vi "Measurement Logic.vi"() -> ()   [LabVIEW 2021, in "Single Tone_Class D Amplifier.lvlib"]
uses:
  Single Tone_Class D Amplifier.lvlib
  Measurement Results.ctl
  <vilib>/PDM Acquisition Toolkit/shared/controls/clock mode.ctl
  <vilib>/PDM Acquisition Toolkit/shared/PDM Shared.lvlib
  <vilib>/PDM Acquisition Toolkit/host/API/PDM Acquisition Toolkit.lvlib
  <vilib>/PDM Acquisition Toolkit/shared/controls/Digital Edge.ctl
  <vilib>/PDM Acquisition Toolkit/shared/controls/PCM Frame Sync Control.ctl
  <vilib>/PDM Acquisition Toolkit/shared/controls/PCM Data Justification.ctl
  <vilib>/PDM Acquisition Toolkit/shared/controls/PCM Bit Endianness.ctl
  <vilib>/PDM Acquisition Toolkit/shared/controls/PCM Data Format Configuration.ctl
  <vilib>/PDM Acquisition Toolkit/host/API/Public/Function Generator/Configure Custom Signal (N Ch) - PCM Output Task.vi
  shared/controls/units - snr.ctl
  shared/controls/audio controls.lvlib
  shared/controls/units - ratio.ctl
  shared/controls/units settings.ctl
  shared/controls/weighting filter.ctl
  shared/controls/highpass filter.ctl
  shared/controls/lowpass filter.ctl
  shared/controls/audio filter settings.ctl
  shared/controls/single tone audio measurement settings.ctl
  shared/controls/digital audio protocol/digital audio protocol controls.lvlib
  <vilib>/Waveform/WDTOps.llb/WDT Get Waveform Subset DBL.vi
  <vilib>/DAQmx/read.llb/DAQmx Read (Analog 1D Wfm NChan NSamp).vi
  <vilib>/DAQmx/configure/timing.llb/DAQmx Timing (Sample Clock).vi
  <vilib>/DAQmx/create/channels.llb/DAQmx Create Channel (AI-Voltage-Basic).vi
  Measurement Configuration.ctl
  <vilib>/MeasurementLink/MeasurementLink Measurement Server/Measure Call Context/Measure Call Context.lvclass
  shared/controls/digital output level units.ctl
  shared/controls/single tone audio measurements.ctl
panel:
  out "names out":string[](array[string])
  out "results":T1[](array[typedef])
  out "Spectrum":cluster{"x0":dbl, "dx":dbl, "magnitude":dbl[]}[](graph)
  out "Waveform Graph":waveform(dbl)[](graph)=[{"t0"=timestamp(3785336549.595634 s since 1904-01-01), "dt"=1.9531249997269942e-05, "Y"=array[12800 elements], "attributes"=variant("NI_ChannelName"=variant(string "PXI1Slot4/ai0"), "NI_UnitDescription"=variant(string "Volts"))}]
  out "Bit Clock Rate":sgl=3072000.0 format="%#_6pHz"
  out "measure call context out":refnum<class "Measure Call Context.lvclass">
  in  "measure call context in":refnum<class "Measure Call Context.lvclass">
  out "measurement results":T2={"channel names"=[], "frequency (Hz)"=[], "amplitude (Vrms)"=[], "amplitude (dBFS)"=[], "phase (deg)"=[], "SNR"=[], "THD+N"=[], "THD"=[], "dynamic range (dB)"=[], "gain"=[], "SFDR (dBc)"=[], "output power (W)"=[], "wfm - t0"=0.0, "wfm - dt"=1.9531249997269942e-05, "wfm - data"=array[12800 elements], "fft - f0"=0.0, "fft - df"=4.000000000559116, "fft - data"=array[6400 elements]}
  in  "measurement configuration":T3={"digital serial cfg file"="", "digital channel list"="7821\\PCMo 8", "master clock channel list"="7821\\PCMo 0", "signal frequency"=1000.0, "output level"=1.0, "output level units"=enum."% FS", "output range (pk-pk)"=15.0, "load impedance"=4.0, "signal phase"=0.0, "acq sampling rate"=51200.0, "min measurement cycles"=20, "min measurement time (s)"=0.1, "min settling cycles"=0, "min settling time (s)"=0.005, "acq channel"="PXI1Slot4/ai0", "band start"=20.0, "band stop"=20000.0, "weighting filter"=enum."Linear", "lowpass filter"=enum."No filter", "highpass filter"=enum."DC", "SNR units"=enum."dB", "THD+N units"=enum."dB", "THD units"=enum."dB", "gain units"=enum."dB"} {"acq sampling rate" format="%#_6p"}
  out "error out":errorcluster
  in  "error in":errorcluster
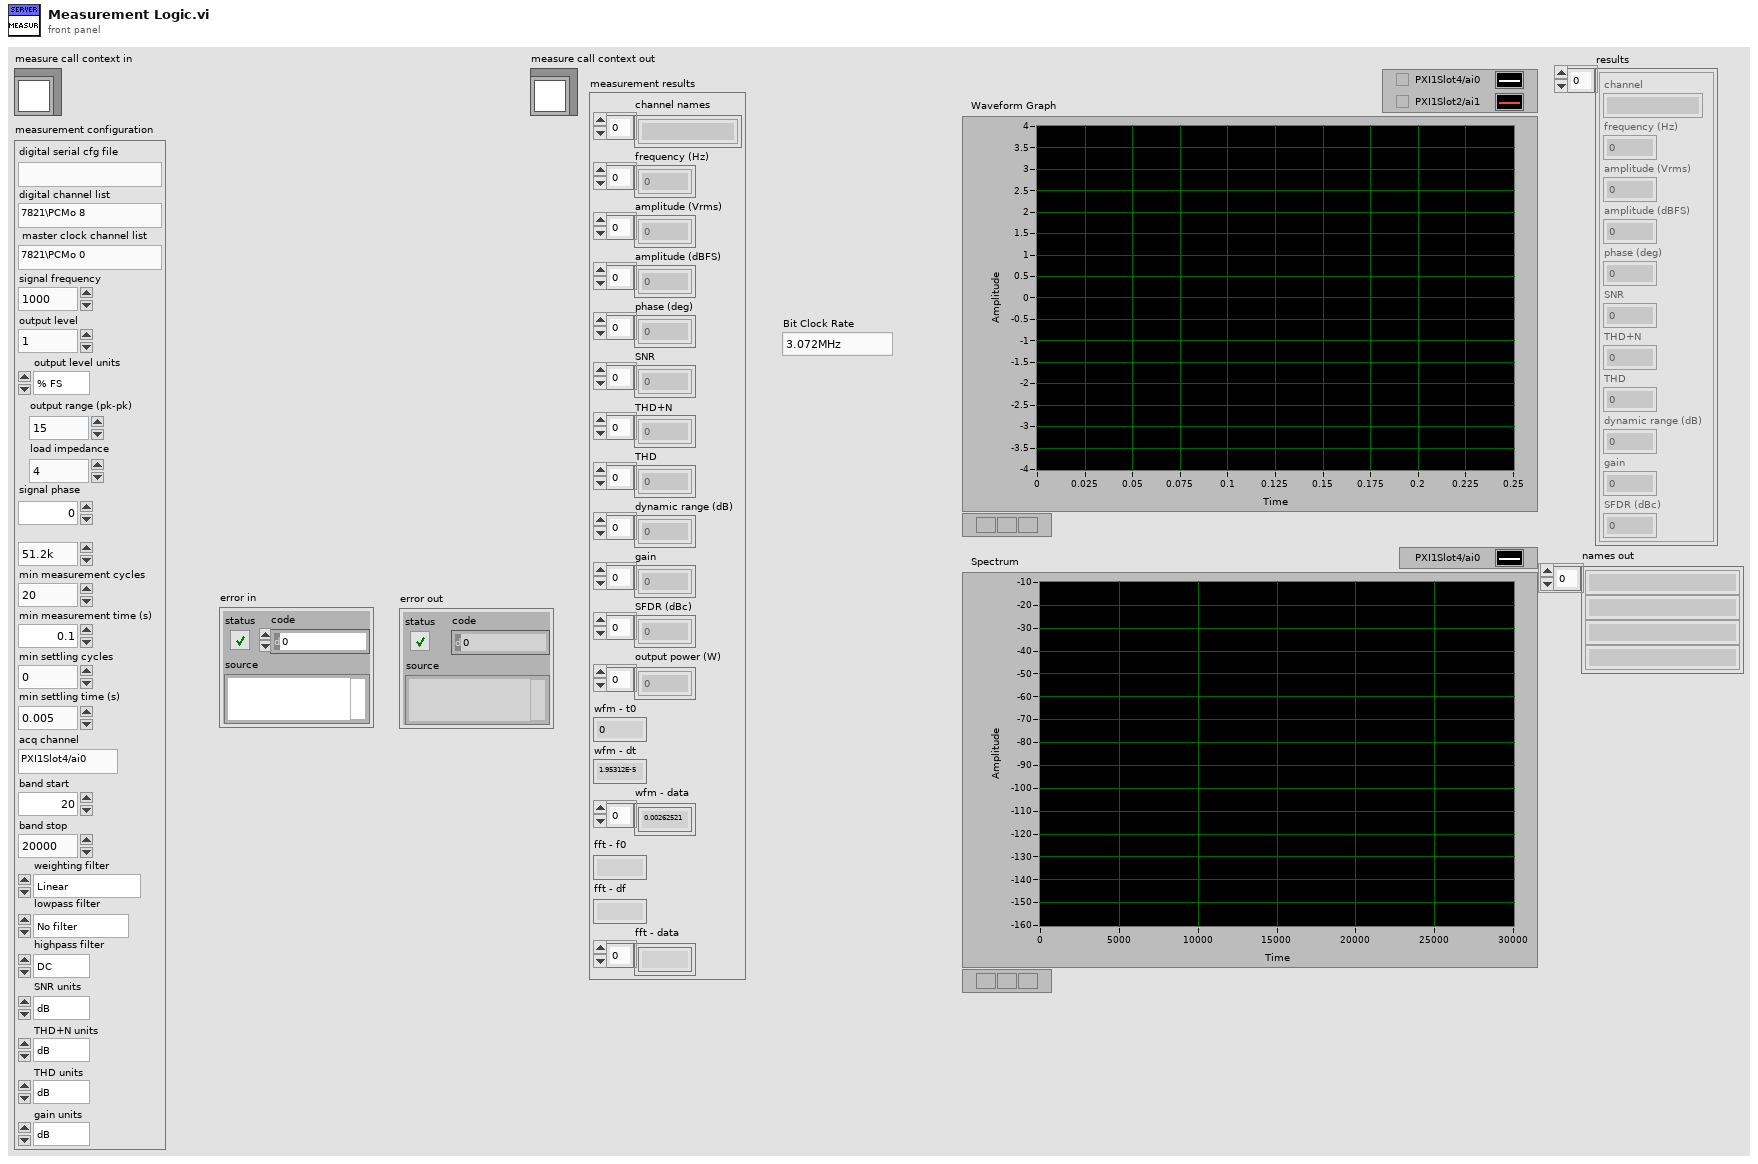
[diagram p1: front panel]
types:
  T1 = typedef "audio controls.lvlib/single tone audio measurements.ctl" = cluster{"channel":string, "frequency (Hz)":dbl, "amplitude (Vrms)":dbl, "amplitude (dBFS)":dbl, "phase (deg)":dbl, "SNR":dbl, "THD+N":dbl, "THD":dbl, "dynamic range (dB)":dbl, "gain":dbl, "SFDR (dBc)":dbl}
  T2 = typedef "Single Tone_Class D Amplifier.lvlib/Measurement Results.ctl" = cluster{"channel names":string[], "frequency (Hz)":dbl[], "amplitude (Vrms)":dbl[], "amplitude (dBFS)":dbl[], "phase (deg)":dbl[], "SNR":dbl[], "THD+N":dbl[], "THD":dbl[], "dynamic range (dB)":dbl[], "gain":dbl[], "SFDR (dBc)":dbl[], "output power (W)":dbl[], "wfm - t0":dbl, "wfm - dt":dbl, "wfm - data":dbl[], "fft - f0":dbl, "fft - df":dbl, "fft - data":dbl[]}
  T3 = typedef "Single Tone_Class D Amplifier.lvlib/Measurement Configuration.ctl" = cluster{"digital serial cfg file":string, "digital channel list":string, "master clock channel list":string, "signal frequency":dbl, "output level":dbl, "output level units":T4, "output range (pk-pk)":dbl, "load impedance":dbl, "signal phase":dbl, "acq sampling rate":dbl, "min measurement cycles":u32, "min measurement time (s)":dbl, "min settling cycles":u32, "min settling time (s)":dbl, "acq channel":string, "band start":dbl, "band stop":dbl, "weighting filter":T5, "lowpass filter":T6, "highpass filter":T7, "SNR units":T8, "THD+N units":T9, "THD units":T9, "gain units":T9}
  T4 = typedef "audio controls.lvlib/digital output level units.ctl" = enum32{"% FS", "dBFS", "V"}
  T5 = typedef "weighting filter.ctl" = enum32{"Linear", "A-weighting", "B-weighting", "C-weighting"}
  T6 = typedef "lowpass filter.ctl" = enum32{"No filter", "AES17 20kHz", "AES17 40kHz"}
  T7 = typedef "highpass filter.ctl" = enum32{"DC", "AC"}
  T8 = typedef "audio controls.lvlib/units - snr.ctl" = enum32{"dB", "x/y"}
  T9 = typedef "audio controls.lvlib/units - ratio.ctl" = enum32{"dB", "%", "x/y"}
  T10 = typedef "audio controls.lvlib/units settings.ctl" = cluster{"SNR units":T8, "THD+N units":T9, "THD units":T9, "gain units":T9}
  T11 = typedef "audio filter settings.ctl" = cluster{"weighting filter":T5, "highpass filter":T7, "lowpass filter ":T6}
  T12 = typedef "single tone audio measurement settings.ctl" = cluster{"Band start":dbl, "Band stop":dbl, "Amplitude":dbl, "Frequency":dbl, "Full scale range":dbl}
  T13 = typedef "PDM Shared.lvlib/PCM Data Format Configuration.ctl" = cluster{"Frame Sync Edge for Channel 0":T14, "Channel Count Per Frame":u8, "Channel Length":u16, "Bit Depth":u8, "Channel 0 Offset":u16, "Endianness":T15, "Data Justification":T16}
  T14 = typedef "PDM Shared.lvlib/Digital Edge.ctl" = enum8{"Rising", "Falling"}
  T15 = typedef "PDM Shared.lvlib/PCM Bit Endianness.ctl" = enum16{"MSB First", "LSB First"}
  T16 = typedef "PDM Shared.lvlib/PCM Data Justification.ctl" = enum16{"Left Justified", "Right Justified"}
  T17 = typedef "PDM Shared.lvlib/PCM Frame Sync Control.ctl" = cluster{"Frame Length":u16, "Frame Sync Pulse Width":u16, "Bit Clock Edge  Sync":T14}
  T18 = typedef "PDM Shared.lvlib/clock mode.ctl" = enum16{"divided clock", "DDS"}
  T19 = typedef "digital audio protocol controls.lvlib/digital audio protocol settings.ctl" = cluster{"number of channels":u32, "data justification":T16, "endianness":T15, "channel length":u32, "bit depth":u32, "frame clock rate":dbl, "bit clock edge sync":T14, "master clock rate":dbl, "Logic Level":T20, "frame sync edge for channel 0":T14, "Channel 0 Offset":u32}
  T20 = typedef "PDM Acquisition Class Library.lvlib/DecoderSession.lvclass/Logic Levels.ctl" = enum16{"3.3 V", "1.8 V", "1.2 V"}
  T21 = typedef "PDM Acquisition Class Library.lvlib/PCM Output Task.lvclass/PCM Output Task DVR.ctl" = refnum<data-value>
  T22 = typedef "PDM Acquisition Class Library.lvlib/I2S Output Task.lvclass/SignalProperties.ctl" = cluster{"cyclic signal":dbl[], "channel parameters":T23[]}
  T23 = typedef "PDM Acquisition Class Library.lvlib/I2S Output Channel.lvclass/GenerationChannelProperties.ctl" = cluster{"cyclic period":dbl, "cyclic phase offset":dbl, "gain":dbl}
  T24 = typedef "audio controls.lvlib/single tone audio measurements (N chan).ctl" = cluster{"channel names":string[], "frequency (Hz)":dbl[], "amplitude (Vrms)":dbl[], "amplitude (dBFS)":dbl[], "phase (deg)":dbl[], "SNR":dbl[], "THD+N":dbl[], "THD":dbl[], "dynamic range (dB)":dbl[], "gain":dbl[], "SFDR (dBc)":dbl[]}
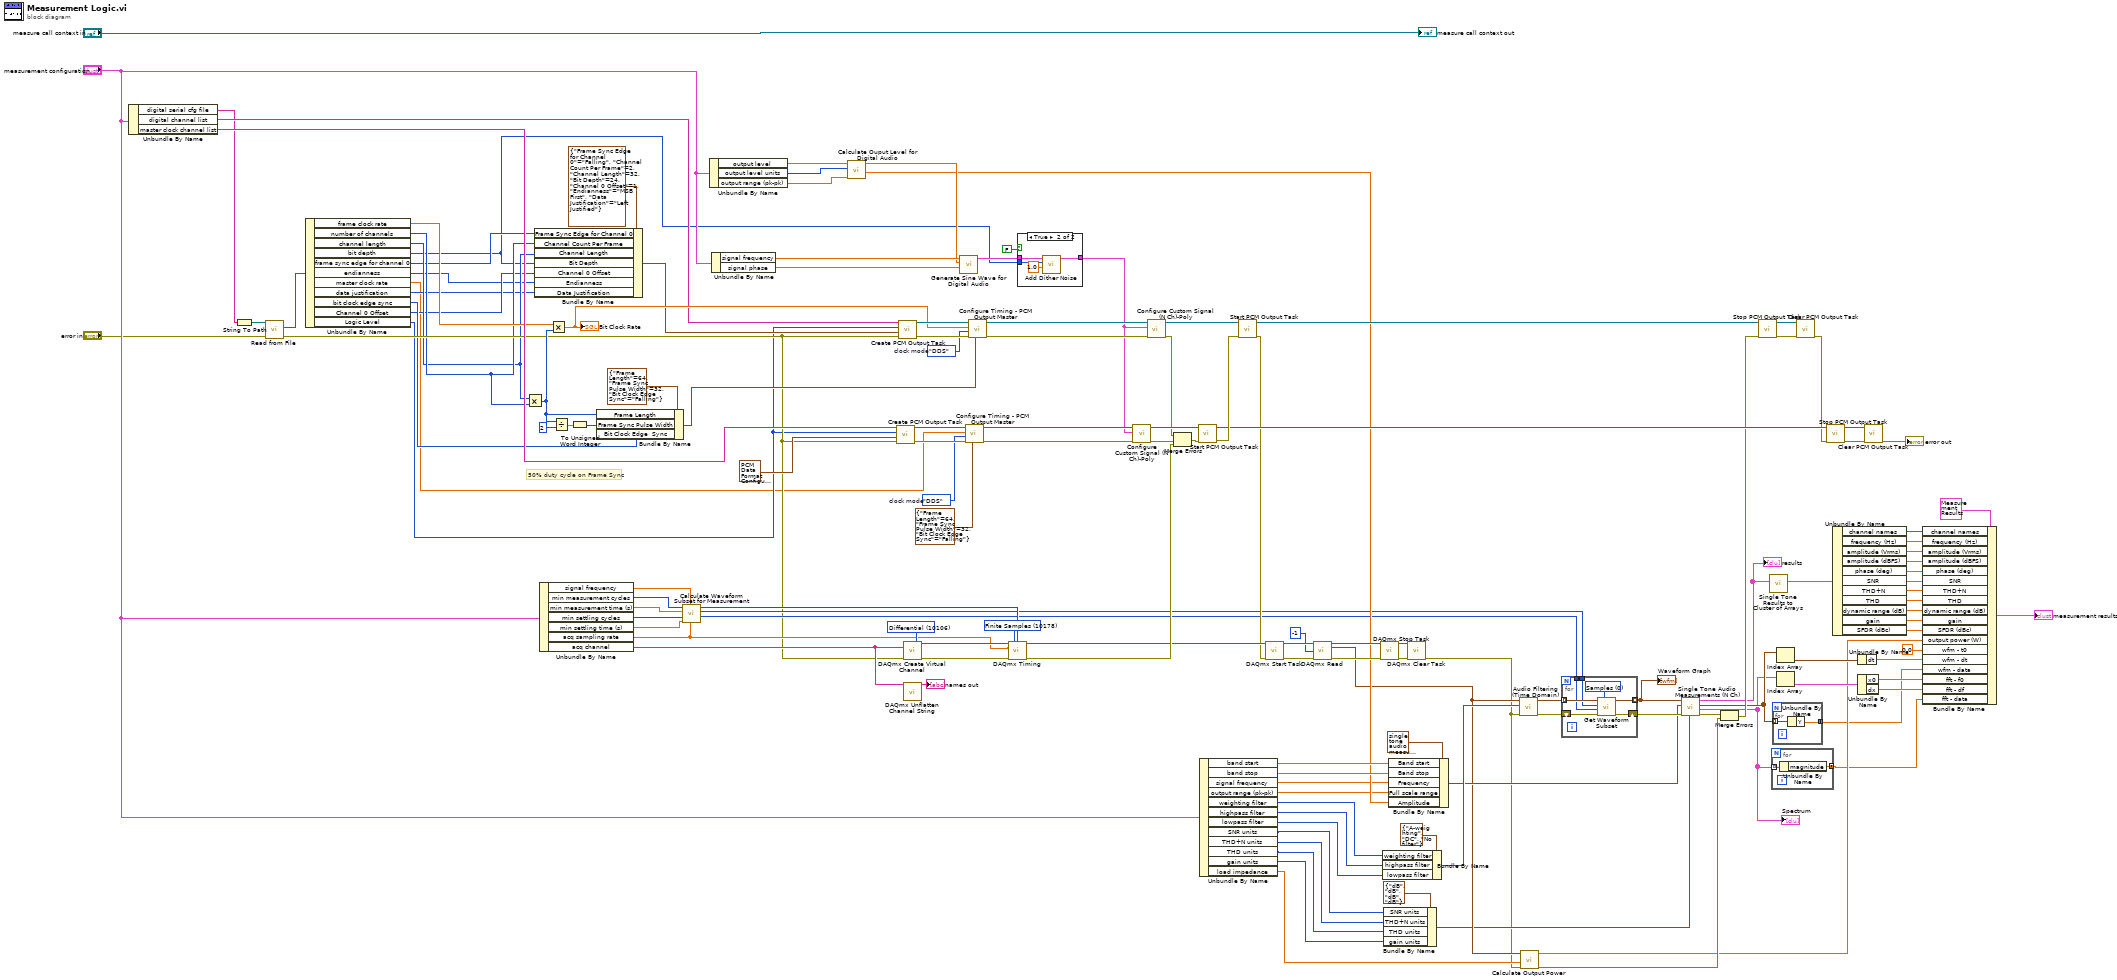
[diagram p0: block diagram]
diagram:
  w93 = 10106 items=["Default"=-1, "RSE"=10083, "NRSE"=10078, "Differential"=10106, "Pseudodifferential"=12529] ("input terminal configuration")
  w99 = 10178 items=["Finite Samples"=10178, "Continuous Samples"=10123, "Hardware Timed Single Point"=12522] ("sample mode")
  w135 = clock_mode."DDS"  # clock mode
  w138 = clock_mode."DDS"  # clock mode
  # "50% duty cycle on Frame Sync"
  n1 = Unbundle By Name("measurement configuration") -> ("digital serial cfg file"=w14:string, "digital channel list"=w66:string, "master clock channel list"=w94:string)
  n2 = String To Path(string=w14) -> (path=w15:path)
  n3 = call "Read from File.vi"("error in (no error)"="error in", "file path"=w15) -> ("error out"=w16:errorcluster, "digital audio protocol settings"=w12:T19)  [unwired: 7 in, 1 out]
  n4 = Unbundle By Name(w12) -> ("frame clock rate"=w11:dbl, "number of channels"=w10:u32, "channel length"=w9:u32, "bit depth"=w1:u32, "frame sync edge for channel 0"=w2:T14, "endianness"=w3:T15, "master clock rate"=w4:dbl, "data justification"=w5:T16, "bit clock edge sync"=w7:T14, "Channel 0 Offset"=w6:u32, "Logic Level"=w8:T20)
  n5 = Multiply(x=w9, y=w10) -> (x*y=w121:u32)
  n6 = Bundle By Name(cluster=T13 {"Frame Sync Edge for Channel 0"=enum."Falling", "Channel Count Per Frame"=2, "Channel Length"=32, "Bit Depth"=24, "Channel 0 Offset"=1, "Endianness"=enum."MSB First", "Data Justification"=enum."Left Justified"} ("PCM Data Configuration"), "Frame Sync Edge for Channel 0"=w2, "Channel Count Per Frame"=w10, "Channel Length"=w9, "Bit Depth"=w1, "Channel 0 Offset"=w6, "Endianness"=w3, "Data Justification"=w5) -> (w118:T13)
  n7 = Unbundle By Name("measurement configuration") -> ("signal frequency"=w58:dbl, "min measurement cycles"=w63:u32, "min measurement time (s)"=w62:dbl, "min settling cycles"=w61:u32, "min settling time (s)"=w60:dbl, "acq sampling rate"=w56:dbl, "acq channel"=w41:string)
  n8 = Multiply(x=w11, y=w121) -> (x*y=w120:dbl)
  "Bit Clock Rate" <- w120
  n9 = Divide(x=w121, y=u16 2) -> (x/y=w123:dbl)
  n10 = To Unsigned Word Integer(number=w123) -> (unsigned 16bit integer=w122:u16)
  n11 = Bundle By Name(cluster=T17 {"Frame Length"=64, "Frame Sync Pulse Width"=32, "Bit Clock Edge  Sync"=enum."Falling"} ("Frame Sync Clock Control"), "Frame Length"=w121, "Frame Sync Pulse Width"=w122, "Bit Clock Edge  Sync"=w7) -> (w125:T17)
  n12 = call "Calculate Waveform Subset for Measurement.vi"("sampling rate"=w56, "signal frequency"=w58, "minimum settling duration"=w60, "minimum settling cycles"=w61, "minimum measurement duration"=w62, "minimum measurement cycles"=w63) -> ("duration (samples)"=w53:u32, "start (samples)"=w54:u32, "total acquisition (samples)"=w55:u32)  [unwired: 3 in]
  n13 = Unbundle By Name("measurement configuration") -> ("output level"=w83:dbl, "output level units"=w82:T4, "output range (pk-pk)"=w81:dbl)
  n14 = Unbundle By Name("measurement configuration") -> ("signal frequency"=w87:dbl, "signal phase"=w91:dbl)
  n15 = call "Calculate Ouput Level for Digital Audio.vi"("output range (pk-pk)"=w81, "digital output level units"=w82, "output level"=w83) -> ("amplitude (pk)"=w67:dbl, "gain"=w86:dbl)  [unwired: 7 in]
  n16 = call <vilib>:"Create PCM Output Task.vi"("error in"=w16, "PCM data configuration"=T13 {"Frame Sync Edge for Channel 0"=enum."Falling", "Channel Count Per Frame"=2, "Channel Length"=32, "Bit Depth"=24, "Channel 0 Offset"=1, "Endianness"=enum."MSB First", "Data Justification"=enum."Left Justified"} ("PCM Data Configuration 2"), "logic level"=w8, "channel list"=w94) -> ("error out"=w136:errorcluster, "PCM output task out"=w137:T21)  [unwired: 6 in]
  n17 = call <vilib>:"Create PCM Output Task.vi"("error in"=w16, "PCM data configuration"=w118, "logic level"=w8, "channel list"=w66) -> ("error out"=w139:errorcluster, "PCM output task out"=w140:T21)  [unwired: 6 in]
  n18 = call-poly <vilib>:"DAQmx Create Virtual Channel.vi"("input terminal configuration"=w93, "physical channels"=w41, "error in"=w16) -> ("task out"=w108:refnum<k21>, "error out"=w109:errorcluster)  [unwired: 11 in]
  n19 = call <vilib>:"DAQmx Unflatten Channel String.vi"("names in"=w41) -> ("names out"=→"names out":string[])  [unwired: 13 in, 1 out]
  n20 = call "Generate Sine Wave for Digital Audio.vi"("phase"=w91, "gain"=w86, "frequency"=w87) -> ("Signal Properties"=w23:T22)  [unwired: 8 in]
  n21 = call <vilib>:"Configure Timing - PCM Output Master.vi"("Frame Sync Clock Control"=T17 {"Frame Length"=64, "Frame Sync Pulse Width"=32, "Bit Clock Edge  Sync"=enum."Falling"} ("Frame Sync Clock Control 2"), "error in"=w136, "clock mode"=w135, "Bit Clock rate"=w4, "PCM output task in"=w137) -> ("error out"=w117:errorcluster, "PCM output task out"=w116:T21)  [unwired: 4 in, 1 out]
  n22 = call <vilib>:"Configure Timing - PCM Output Master.vi"("Frame Sync Clock Control"=w125, "error in"=w139, "clock mode"=w138, "Bit Clock rate"=w120, "PCM output task in"=w140) -> ("error out"=w84:errorcluster, "PCM output task out"=w85:T21)  [unwired: 4 in, 1 out]
  n23 = call-poly <vilib>:"DAQmx Timing.vi"("task/channels in"=w108, "sample mode"=w99, "samples per channel"=w55, "rate"=w56, "error in"=w109) -> ("task out"=w100:refnum<k21>, "error out"=w101:errorcluster)  [unwired: 9 in]
  n24 = case shown="True" FALSE {
    tunnel: w23 -> [w144 w148]
    tunnel: [w144 w147] -> w22
    tunnel: w1 -> [_ w146]
    frame False {
    }
    frame True {
      n25 = call "Add Dither Noise.vi"("amplitude (LSB)"=1.0, "bits"=w146, "Signal Properties"=w148) -> ("Signal Properties"=w147:T22)  [unwired: 8 in]
    }
  }
  n26 = call-poly <vilib>:"Configure Custom Signal (N Ch)-Poly.vi"("error in"=w117, "signal parameters"=w22, "PCM output task in"=w116) -> ("error out"=w112:errorcluster, "PCM output task out"=w115:T21)  [unwired: 7 in]
  n27 = call-poly <vilib>:"Configure Custom Signal (N Ch)-Poly.vi"("error in"=w84, "signal parameters"=w22, "PCM output task in"=w85) -> ("error out"=w113:errorcluster, "PCM output task out"=w114:T21)  [unwired: 7 in]
  n28 = Merge Errors(w113, w112, w101) -> (w131:errorcluster)
  n29 = call <vilib>:"Start PCM Output Task.vi"("error in"=w131, "PCM output task in"=w115) -> ("error out"=w132:errorcluster, "PCM output task out"=w128:T21)  [unwired: 8 in]
  n30 = Unbundle By Name("measurement configuration") -> ("band start"=w75:dbl, "band stop"=w74:dbl, "signal frequency"=w64:dbl, "output range (pk-pk)"=w65:dbl, "weighting filter"=w72:T5, "highpass filter"=w71:T7, "lowpass filter"=w70:T6, "SNR units"=w49:T8, "THD+N units"=w48:T9, "THD units"=w47:T9, "gain units"=w46:T9, "load impedance"=w50:dbl)
  n31 = call <vilib>:"Start PCM Output Task.vi"("error in"=w132, "PCM output task in"=w114) -> ("error out"=w92:errorcluster, "PCM output task out"=w111:T21)  [unwired: 8 in]
  n32 = call <vilib>:"DAQmx Start Task.vi"("task/channels in"=w100, "error in"=w92) -> ("task out"=w103:refnum<k21>, "error out"=w106:errorcluster)  [unwired: 12 in]
  n33 = call-poly <vilib>:"DAQmx Read.vi"("task/channels in"=w103, "number of samples per channel"=-1, "error in"=w106) -> ("task out"=w102:refnum<k21>, "data"=w57:waveform(dbl)[], "error out"=w105:errorcluster)  [unwired: 10 in]
  n34 = call <vilib>:"DAQmx Stop Task.vi"("task/channels in"=w102, "error in"=w105) -> ("task out"=w107:refnum<k21>, "error out"=w104:errorcluster)  [unwired: 12 in]
  n35 = Bundle By Name(cluster=T11 {"weighting filter"=enum."A-weighting", "highpass filter"=enum."DC", "lowpass filter "=enum."No filter"} ("filter settings"), "weighting filter"=w72, "highpass filter"=w71, "lowpass filter"=w70) -> (w69:T11)
  n36 = Bundle By Name(cluster=T10 {"SNR units"=enum."dB", "THD+N units"=enum."dB", "THD units"=enum."dB", "gain units"=enum."dB"} ("units settings"), "SNR units"=w49, "THD+N units"=w48, "THD units"=w47, "gain units"=w46) -> (w51:T10)
  n37 = Bundle By Name(cluster=T12 {"Band start"=20.0, "Band stop"=20000.0, "Amplitude"=-1.0, "Frequency"=1000.0, "Full scale range"=15.0} ("measurement settings"), "Band start"=w75, "Band stop"=w74, "Frequency"=w64, "Full scale range"=w65, "Amplitude"=w67) -> (w68:T12)
  n38 = call <vilib>:"DAQmx Clear Task.vi"("task in"=w107, "error in"=w104) -> ("error out"=w45:errorcluster)  [unwired: 13 in]
  n39 = call "Audio Filtering (Time Domain).vi"("waveforms"=w57, "filter settings"=w69, "error in"=w45) -> ("time domain"=w79:waveform(dbl)[], "error out"=w80:errorcluster)  [unwired: 6 in]
  n40 = call "Calculate Output Power.vi"("error in (no error)"=w45, "load impedance"=w50, "waveforms"=w57) -> ("error out"=w88:errorcluster, "output power"=w24:dbl[])  [unwired: 7 in]
  n41 = for {
    tunnel: w79 -> [w155] mode=indexing
    tunnel: [w154] -> w44 mode=indexing
    shift-right: [w151] -> w78
    shift-left: w80 -> [w152]
    tunnel: w54 -> [w150]
    tunnel: w53 -> [w149]
    w153 = u16 0 items=["Samples", "Relative Time"] ("start/duration format")
    n42 = call-poly <vilib>:"Get Waveform Subset.vi"("start/duration format"=w153, "error in (no error)"=w152, "duration"=w149, "start samples/time"=w150, "waveform in"=w155) -> ("error out"=w151:errorcluster, "waveform out"=w154:waveform(dbl))  [unwired: 1 in, 2 out]
  }
  "Waveform Graph" <- w44
  n43 = call "Single Tone Audio Measurements (N Ch).vi"("units settings"=w51, "error in"=w78, "measurement settings"=w68, "waveforms"=w44) -> ("error out"=w77:errorcluster, "spectra"=w20:cluster{"x0":dbl, "dx":dbl, "magnitude":dbl[]}[], "waveforms"=w21:waveform(dbl)[], "results"=w37:T1[])  [unwired: 4 in]
  "Spectrum" <- w20
  "results" <- w37
  n44 = Merge Errors(w77, w88) -> (w89:errorcluster)
  n45 = call <vilib>:"Stop PCM Output Task.vi"("error in"=w89, "PCM output task In"=w111) -> ("error out"=w142:errorcluster, "PCM output task out"=w141:T21)  [unwired: 8 in]
  n46 = call "Single Tone Results to Cluster of Arrays.vi"("results"=w37) -> ("results (N chan)"=w36:T24)  [unwired: 10 in]
  n47 = for {
    tunnel: w20 -> [w157] mode=indexing
    tunnel: [w156] -> w19 mode=concatenating
    n48 = Unbundle By Name(w157) -> ("magnitude"=w156:dbl[])
  }
  n49 = for {
    tunnel: w21 -> [w159] mode=indexing
    tunnel: [w158] -> w18 mode=concatenating
    n50 = Unbundle By Name(w159) -> ("Y"=w158:dbl[])
  }
  n51 = Index Array(array=w21) -> (element=w43:waveform(dbl))  [unwired: 1 in]
  n52 = Index Array(array=w20) -> (element=w42:cluster{"x0":dbl, "dx":dbl, "magnitude":dbl[]})  [unwired: 1 in]
  n53 = call <vilib>:"Clear PCM Output Task.vi"("error in"=w142, "PCM output task in"=w141) -> ("error out"=w127:errorcluster)  [unwired: 9 in]
  n54 = call <vilib>:"Stop PCM Output Task.vi"("error in"=w127, "PCM output task In"=w128) -> ("error out"=w130:errorcluster, "PCM output task out"=w129:T21)  [unwired: 8 in]
  n55 = Unbundle By Name(w36) -> ("channel names"=w35:string[], "frequency (Hz)"=w34:dbl[], "amplitude (Vrms)"=w33:dbl[], "amplitude (dBFS)"=w32:dbl[], "phase (deg)"=w31:dbl[], "SNR"=w30:dbl[], "THD+N"=w29:dbl[], "THD"=w28:dbl[], "dynamic range (dB)"=w27:dbl[], "gain"=w26:dbl[], "SFDR (dBc)"=w25:dbl[])
  n56 = Unbundle By Name(w43) -> ("dt"=w97:dbl)
  n57 = Unbundle By Name(w42) -> ("x0"=w96:dbl, "dx"=w95:dbl)
  n58 = call <vilib>:"Clear PCM Output Task.vi"("error in"=w130, "PCM output task in"=w129) -> ("error out"=→"error out":errorcluster)  [unwired: 9 in]
  n59 = Bundle By Name(cluster=T2 {"channel names"=[], "frequency (Hz)"=[], "amplitude (Vrms)"=[], "amplitude (dBFS)"=[], "phase (deg)"=[], "SNR"=[], "THD+N"=[], "THD"=[], "dynamic range (dB)"=[], "gain"=[], "SFDR (dBc)"=[], "output power (W)"=[], "wfm - t0"=0.0, "wfm - dt"=0.0, "wfm - data"=[], "fft - f0"=0.0, "fft - df"=0.0, "fft - data"=[]} ("Measurement Results"), "channel names"=w35, "frequency (Hz)"=w34, "amplitude (Vrms)"=w33, "amplitude (dBFS)"=w32, "phase (deg)"=w31, "SNR"=w30, "THD+N"=w29, "THD"=w28, "dynamic range (dB)"=w27, "gain"=w26, "SFDR (dBc)"=w25, "output power (W)"=w24, "wfm - t0"=0.0, "wfm - dt"=w97, "wfm - data"=w18, "fft - f0"=w96, "fft - df"=w95, "fft - data"=w19) -> (→"measurement results":T2)
  "measure call context out" <- "measure call context in"
